vi "tm_setparameter_40.vi"(6 "Index":i32, 7 "Reconfigure (F)":bool, 8 "error in (no error)":errorcluster, 9 "Value in":dbl, 10 "Parameter":u32(ring)=4212128 items=["SENSOR MODE"=4212128, "SENSOR MODE LINE BUNDLE HEIGHT"=4212192, "READOUT DIRECTION"=4211904, "BIT PER CHANNEL"=4342976, "EXPOSURE TIME"=2049184, "CONTRAST GAIN"=3163312, "BINNING"=4215968, "TIMING READOUT TIME"=4223904, "INTERNAL FRAME RATE"=4225952, "INTERNAL FRAME INTERVAL"=4225968, "INTERNAL LINE SPEED"=4226000, "IMAGE WIDTH"=4343200, "IMAGE HEIGHT"=4343216, "IMAGE ROWBYTES"=4343232, "IMAGE FRAMEBYTES"=4343248, "IMAGE PIXEL TYPE"=4343296], 11 "Handle in":u32) -> (0 "error out":errorcluster, 3 "Handle out":u32)   [LabVIEW 2023]
uses:
  tmcamcon.dll
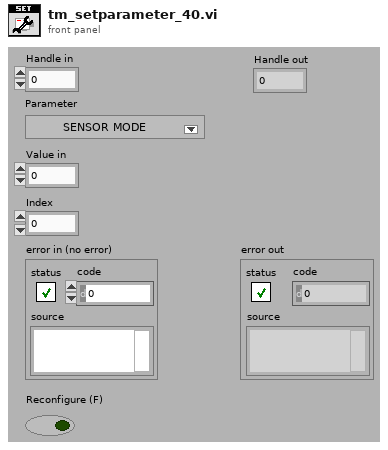
[diagram p1: front panel]
types:
  T1 = cluster{"Property Name":string, "Property ID":i32}[]
  T2 = cluster{"Property Name":string, "Property ID":i32}
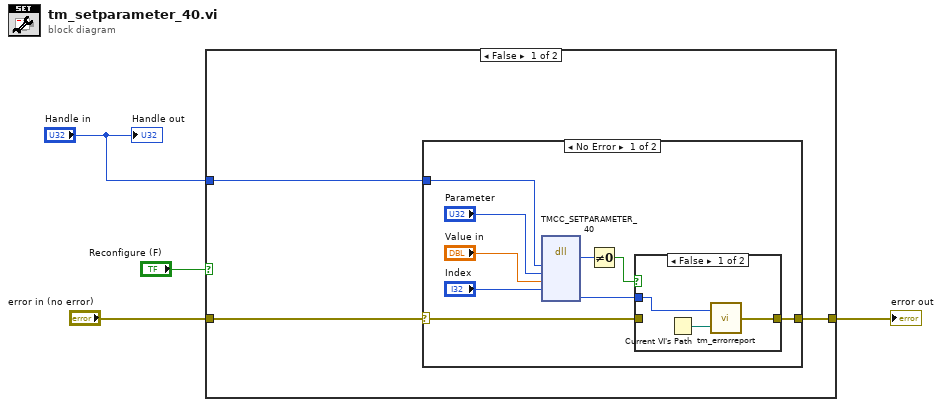
[diagram p0: block diagram]
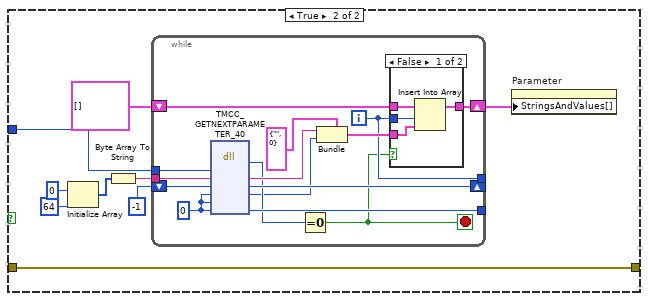
[diagram p4: hidden frame]
diagram:
  n1 = case shown="False" "Reconfigure (F)" {
    tunnel: "error in (no error)" -> [w6 w30]
    tunnel: [w7 w30] -> w2
    tunnel: "Handle in" -> [w5 w22]
    frame False {
      n2 = case shown="No Error" w6 {
        selector: w6 -> [w11 w21]
        tunnel: [w8 w21] -> w7
        tunnel: w5 -> [w12 _]
        frame No Error {
          n3 = dll-call lib="tmcamcon.dll" fn="TMCC_SETPARAMETER_40"("HDCAM"=w12, "parameter"="Parameter", "value"="Value in", "view"="Index") -> ("return type"=w16:u32, "Erval"=w10:i32)  [unwired: 8 in, 2 out]
          n4 = Not Equal To 0?(x=w16) -> (x != 0?=w9:bool)
          n5 = case shown="False" w9 {
            tunnel: w11 -> [_ w20]
            tunnel: [w18 w20] -> w8
            tunnel: w10 -> [w17 _]
            frame False {
              n6 = Current VI's Path() -> (path=w19:path)
              n7 = call "tm_errorreport.vi"("Source"=w19, "Error"=w17) -> ("error out"=w18:errorcluster)
            }
            frame True {
            }
          }
        }
        frame Error {
        }
      }
    }
    frame True {
      n8 = Initialize Array(u8 0 ("element"), 64 ("dimension size")) -> (w28:u8[])
      n9 = Byte Array To String(unsigned byte array=w28) -> (string=w25:string)
      n10 = while {
        shift-right: [w44] -> w23
        shift-left: T1 [] ("Array") -> [w45]
        tunnel: [w40] -> _
        tunnel: [w38] -> _
        tunnel: w25 -> [w37]
        tunnel: w22 -> [w36]
        shift-right: [w39] -> _
        shift-left: -1 ("func_num") -> [w41]
        i -> [w38]
        stop <- w34 stop-if-true
        w31 = 0 ("option")
        n11 = dll-call lib="tmcamcon.dll" fn="TMCC_GETNEXTPARAMETER_40"("HDCAM"=w36, "name"=w37, "func_num"=w41, "func_id"=w31, "option"=w31, "Erval"=w31) -> ("return type"=w33:u32, "name"=w42:string, "func_num"=w39:i32, "func_id"=w32:i32, "Erval"=w40:i32)  [unwired: 5 in, 2 out]
        n12 = Equal To 0?(x=w33) -> (x = 0?=w34:bool)
        n13 = Bundle(cluster=T2 {"Property Name"="", "Property ID"=0} ("new element/subarray"), "Property Name"=w42, "Property ID"=w32) -> (w43:T2)
        n14 = case shown="False" w34 {
          tunnel: w45 -> [w49 w50]
          tunnel: [w48 w50] -> w44
          tunnel: w38 -> [w47 _]
          tunnel: w43 -> [w46 _]
          frame False {
            n15 = Insert Into Array(array=w49, index=w47, new element=w46) -> (w48:T1)
          }
          frame True {
          }
        }
      }
      n16 = property on="Parameter" class="Ring (strict)"("StringsAndValues[]"=w23) -> ()  [unwired: 2 in, 2 out]
    }
  }
  "error out" <- w2
  "Handle out" <- "Handle in"
